vi "Capture Event.vi"(7 "event # to capture":T3=1, 10 "measured data":T2) -> (3 "capture.<user name>":T1)   [LabVIEW 2013, in "Engine Simulation Toolkit.lvlib" / "ECU Event Timing.lvlib"]
doc: "Latches event measurement data for a particular event (pulse) into an indicator for NI VeriStand to read. \n\n<b>event # to capture</b> - the event (pulse) number to latch data from, in a sequence of events (pulses). For example, a value of 2 means latch the 2nd event's data into the indicator.\n<b>measured data</b> - event measurement data coming from Measure Event.vi\n\n<b>capture.<user name></b> - output for the component. NI VeriStand will read these values. Create an indicator for this output. Replace <user name> with the name you wish this component to display as inside NI VeriStand. Make this name consistent for all controls, indicators, for all VIs of this component."
uses:
  ECU Event Timing.lvlib
  Capture Settings.ctl
  Measured Data.ctl
  Capture Output.ctl
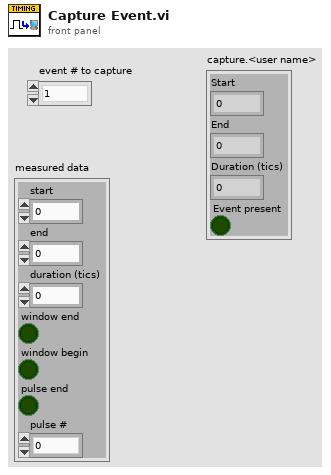
[diagram p1: front panel]
types:
  T1 = typedef "Engine Simulation Toolkit.lvlib/ECU Event Timing.lvlib/Capture Output.ctl" = cluster{"Start":u16, "End":u16, "Duration (tics)":fxp<+,18,18>, "Event present":bool}
  T2 = typedef "Engine Simulation Toolkit.lvlib/ECU Event Timing.lvlib/Measured Data.ctl" = cluster{"start":u16, "end":u16, "duration (tics)":fxp<+,18,18>, "window end":bool, "window begin":bool, "pulse end":bool, "pulse #":u8}
  T3 = typedef "Engine Simulation Toolkit.lvlib/ECU Event Timing.lvlib/Capture Settings.ctl" = u8
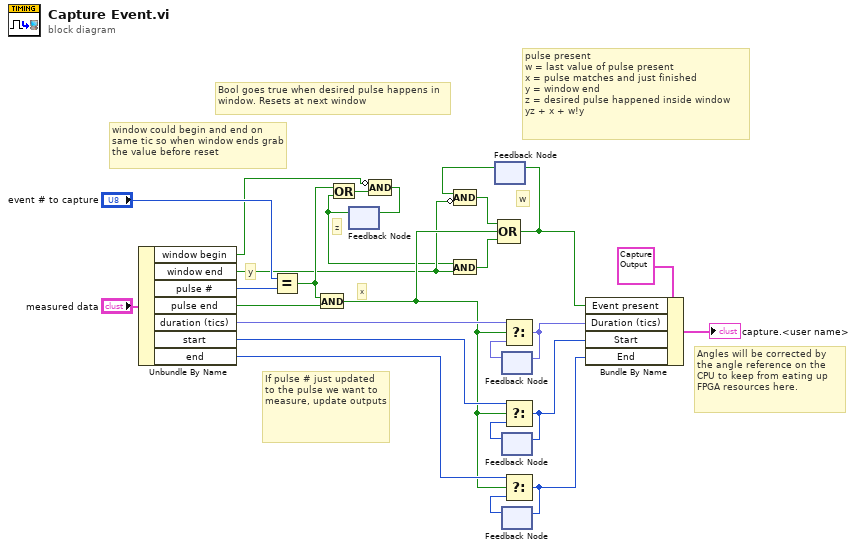
[diagram p0: block diagram]
diagram:
  # "window could begin and end on same tic so when window ends grab the value before reset"
  # "w"
  # "pulse present\nw = last value of pulse present\nx = pulse matches and just finished\ny = window end\nz = desired pulse happened inside window\nyz + x + w!y"
  # "z"
  # "y"
  # "x"
  # "Angles will be corrected by the angle reference on the CPU to keep from eating up FPGA resources here."
  # "Bool goes true when desired pulse happens in window. Resets at next window"
  # "If pulse # just updated to the pulse we want to measure, update outputs"
  n1 = Unbundle By Name("measured data") -> ("window begin"=w9:bool, "window end"=w3:bool, "pulse #"=w21:u8, "pulse end"=w22:bool, "duration (tics)"=w16:fxp<+,18,18>, "start"=w19:u16, "end"=w17:u16)
  n2 = Equal?(x="event # to capture", y=w21) -> (x = y?=w26:bool)
  n3 = And(x=w26, y=w22) -> (x .and. y?=w4:bool)
  n4 = feedback #1() -> (w1:bool)  [unwired: 1 in]
  n5 = Or(x=w26, y=w1) -> (x .or. y?=w25:bool)
  n6 = Compound Arithmetic op=AND(invert w9, w25) -> (w2:bool)
  n7 = feedback-in #1(w2) -> ()
  n8 = And(x=w1, y=w3) -> (x .and. y?=w6:bool)
  n9 = feedback #2() -> (w5:bool)  [unwired: 1 in]
  n10 = Compound Arithmetic op=AND(w5, invert w3) -> (w7:bool)
  n11 = Compound Arithmetic op=OR(w7, w4, w6) -> (w8:bool)
  n12 = feedback-in #2(w8) -> ()
  n13 = feedback #3() -> (w15:fxp<+,18,18>)  [unwired: 1 in]
  n14 = feedback #4() -> (w20:u16)  [unwired: 1 in]
  n15 = feedback #5() -> (w18:u16)  [unwired: 1 in]
  n16 = Select(t=w16, s=w4, f=w15) -> (s? t:f=w12:fxp<+,18,18>)
  n17 = feedback-in #3(w12) -> ()
  n18 = Select(t=w19, s=w4, f=w20) -> (s? t:f=w11:u16)
  n19 = feedback-in #4(w11) -> ()
  n20 = Select(t=w17, s=w4, f=w18) -> (s? t:f=w10:u16)
  n21 = feedback-in #5(w10) -> ()
  n22 = Bundle By Name(cluster=T1 {"Start"=0, "End"=0, "Duration (tics)"=0.0, "Event present"=FALSE} ("output"), "Event present"=w8, "Duration (tics)"=w12, "Start"=w11, "End"=w10) -> (→"capture.<user name>":T1)
